vi "test realtime main.vi"() -> ()   [LabVIEW 2012]
panel:
  in  "Average N Reference Frames":dbl=1.0 min=1.0
  in  "Position Shift Limit (Microns)":dbl=3.0 min=0.0
  out "Out of Limits":bool
  in  "output cluster":T1
  out "Z":dbl(graph)
  out "Y":dbl(graph)
  out "X":dbl(graph)
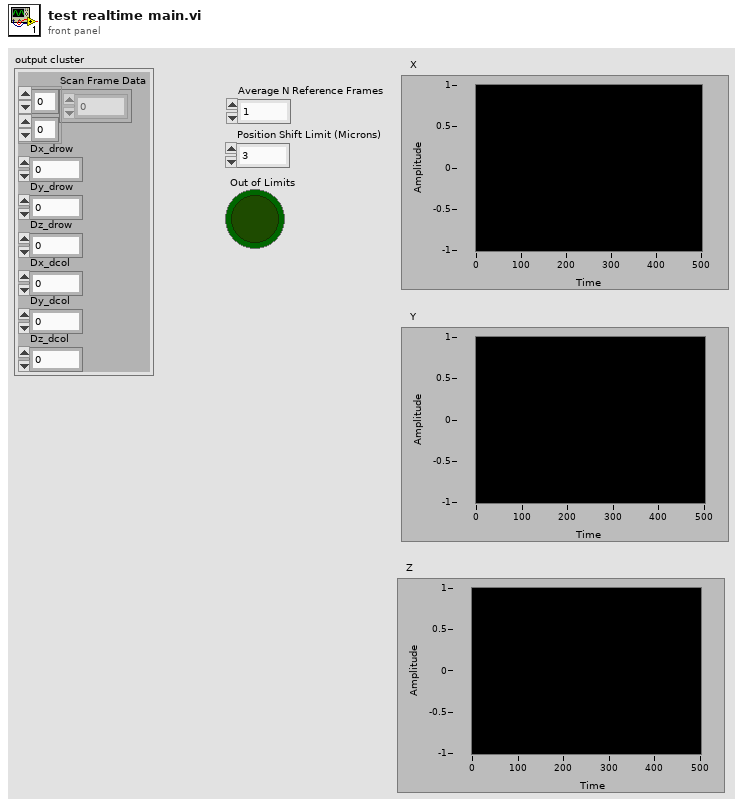
[diagram p1: front panel]
types:
  T1 = cluster{"Scan Frame Data":dbl[][], "Dx_drow":dbl, "Dy_drow":dbl, "Dz_drow":dbl, "Dx_dcol":dbl, "Dy_dcol":dbl, "Dz_dcol":dbl}
  T2 = cluster{"PMTChans":i32, "NumScanPlanes":i32, "ScanRows":i32, "ScanCols":i32, "NumSamples":i32}
  T3 = cluster{"Scan Frame Data":dbl[][], "Dx_drow":dbl, "Dy_drow":dbl, "Dz_drow":dbl, "Dx_dcol":dbl, "Dy_dcol":dbl, "Dz_dcol":dbl}[]
  T4 = cluster{"Scan Frame Data":dbl[][], dbl, dbl, dbl, dbl, dbl, dbl}
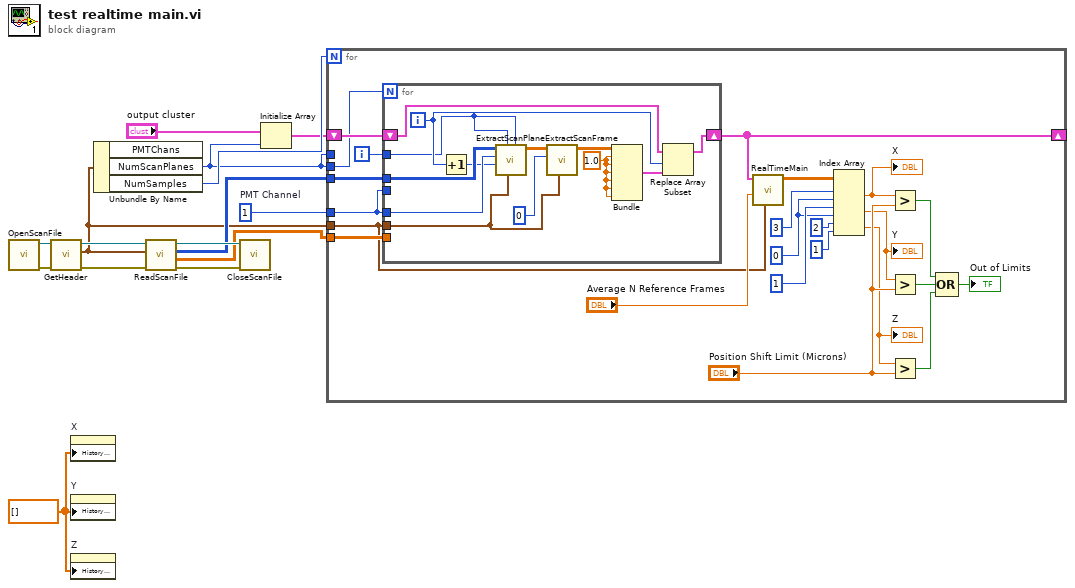
[diagram p0: block diagram]
diagram:
  w2 = dbl[] [] ("History Data")
  w6 = 1  # PMT Channel
  n1 = call "OpenScanFile.vi"() -> ("error out"=w14:errorcluster, "refnum out"=w15:refnum<file>)  [unwired: 10 in]
  n2 = call "GetHeader.vi"("error in"=w14, "refnum in"=w15) -> ("error out"=w10:errorcluster, "Header"=w7:T2, "refnum out"=w13:refnum<file>)  [unwired: 6 in]
  n3 = property on="X" class="WFChart (strict)"("History Data"=w2) -> ()  [unwired: 2 in, 2 out]
  n4 = property on="Y" class="WFChart (strict)"("History Data"=w2) -> ()  [unwired: 2 in, 2 out]
  n5 = property on="Z" class="WFChart (strict)"("History Data"=w2) -> ()  [unwired: 2 in, 2 out]
  n6 = Unbundle By Name(w7) -> ("NumScanPlanes"=w1:i32, "NumSamples"=w5:i32)  [unwired: 1 out]
  n7 = call "ReadScanFile.vi"("error in"=w10, "Header"=w7, "refnum in"=w13) -> ("error out"=w11:errorcluster, "Coordinate Data"=w8:dbl[][][][], "Scan Data"=w9:i32[][][][], "refnum out"=w12:refnum<file>)  [unwired: 5 in]
  n8 = call "CloseScanFile.vi"("error in"=w11, "refnum"=w12) -> ()  [unwired: 9 in, 1 out]
  n9 = Initialize Array("output cluster", w1) -> (w3:T3)
  n10 = for {
    N: w5 -> [_]
    tunnel: w9 -> [w38]
    tunnel: w8 -> [w37]
    tunnel: w7 -> [w16]
    tunnel: w1 -> [w33]
    tunnel: w6 -> [w36]
    shift-right: [w32] -> _
    shift-left: w3 -> [w34]
    tunnel: w1 -> [_]
    i -> [w35]
    w27 = 0 ("disabled index (col)")
    n11 = for {
      N: w33 -> [_]
      tunnel: w38 -> [w51]
      tunnel: w36 -> [w50]
      tunnel: w37 -> [_]
      tunnel: w16 -> [w47]
      tunnel: w36 -> [_]
      tunnel: w35 -> [w41]
      shift-right: [w42] -> w32
      shift-left: w34 -> [w45]
      i -> [w43]
      w39 = 1.0
      n12 = Increment(x=w43) -> (x+1=w48:i32)
      n13 = call "ExtractScanPlane.vi"("End Frame"=w41, "Header"=w47, "Start Frame"=w41, "Scan Plane"=w48, "PMT Channel"=w50, "All Scan Data"=w51) -> ("Scan Plane Data"=w49:dbl[][][])  [unwired: 5 in]
      n14 = call "ExtractScanFrame.vi"("Header"=w47, "Scan Frame"=0, "Scan Plane Data"=w49) -> ("Scan Frame Data"=w46:dbl[][])  [unwired: 8 in]
      n15 = Bundle("Scan Frame Data"=w46, w39, w39, w39, w39, w39, w39) -> (w44:T4)  [unwired: 1 in]
      n16 = Replace Array Subset(array=w45, new element=w44, index=w43) -> (w42:T3)
    }
    n17 = call "RealTimeMain.vi"("Header"=w16, "For Reference (frames)"="Average N Reference Frames", "Motion Data"=w32) -> ("Array"=w22:dbl[][])  [unwired: 8 in]
    n18 = Index Array(array=w22, index (row) #1=3 ("index (row)"), index (col) #1=w27, index (row) #2=1 ("index (row)"), index (col) #2=w27, index (row) #3=2 ("index (row)"), index (col) #3=1 ("disabled index (col)")) -> (element #1=w19:dbl, element #2=w18:dbl, element #3=w17:dbl)
    "X" <- w19
    "Y" <- w18
    "Z" <- w17
    n19 = Greater?(x=w19, y="Position Shift Limit (Microns)") -> (0:w25:bool)
    n20 = Greater?(x=w18, y="Position Shift Limit (Microns)") -> (0:w24:bool)
    n21 = Greater?(x=w17, y="Position Shift Limit (Microns)") -> (0:w23:bool)
    n22 = Compound Arithmetic op=OR(w25, w24, w23) -> (→"Out of Limits":bool)
  }
